vi "nanostage-init.vi"(3 "error in":errorcluster, 4 "Perform autozero?":bool=TRUE) -> (0 "error out":errorcluster, 2 "All conn. axes":string[](array[string]))   [LabVIEW 2017]
panel:
  out "USB: S/N out":string
  # "3D piezo nano stage"
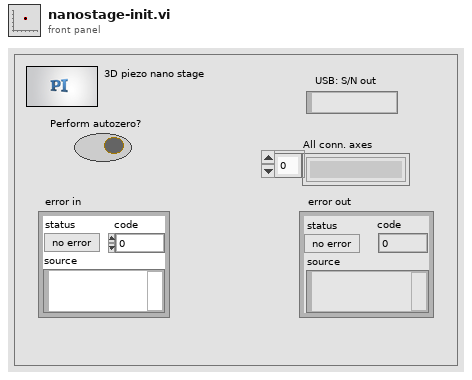
[diagram p1: front panel]
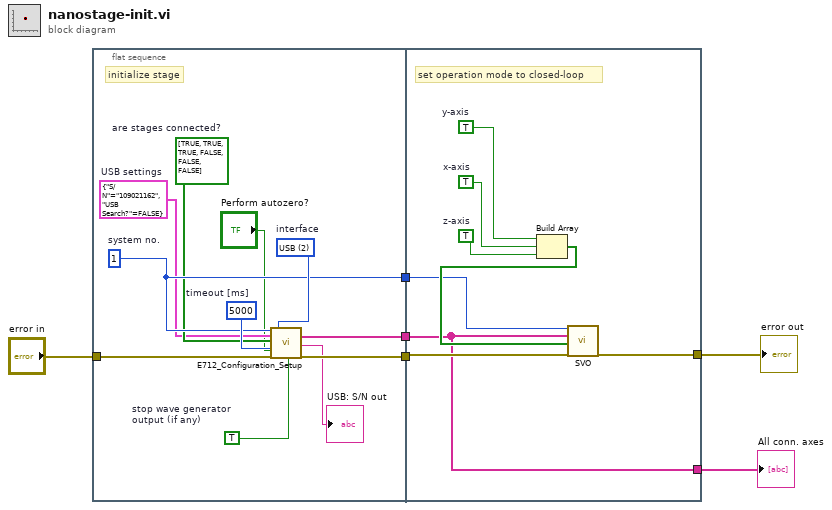
[diagram p0: block diagram]
diagram:
  n1 = flat-sequence {
    tunnel: [w15] -> w5
    tunnel: [w14] -> w4
    tunnel: [w9] -> w3
    tunnel: "error in" -> [w11]
    tunnel: w5 -> [w20]
    tunnel: w4 -> [w18]
    tunnel: w3 -> [w25]
    tunnel: [w19] -> w2
    tunnel: [w18] -> w1
    frame #0 {
      w10 = cluster{"S/N":string, "USB Search?":bool} {"S/N"="109021162", "USB Search?"=FALSE}  # USB settings
      w12 = bool[] [TRUE, TRUE, TRUE, FALSE, FALSE, FALSE]  # are stages connected?
      w13 = TRUE  # stop wave generator output (if any)
      w16 = 5000  # timeout [ms]
      w15 = 1  # system no.
      w17 = u16 2 items=["RS232", "TCP/IP", "USB"]  # interface
      # "initialize stage"
      n2 = call "E712_Configuration_Setup.vi"("System no."=w15, "USB settings"=w10, "Are stages connected?"=w12, "Perform autozero?"="Perform autozero?", "error in"=w11, "Interface"=w17, "Timeout"=w16, "Stop wave generator\noutput (if any)"=w13) -> ("All conn. axes"=w14:string[], "USB: S/N out"=→"USB: S/N out":string, "error out"=w9:errorcluster)  [unwired: 7 in, 2 out]
    }
    frame #1 {
      w21 = TRUE  # z-axis
      w22 = TRUE  # x-axis
      w23 = TRUE  # y-axis
      # "set operation mode to closed-loop"
      n3 = Build Array(w23, w22, w21) -> (w24:bool[])
      n4 = call "SVO.vi"("System no."=w20, "Axes to command"=w18, "Servo mode"=w24, "error in"=w25) -> ("error out"=w19:errorcluster)  [unwired: 15 in]
    }
  }
  "error out" <- w2
  "All conn. axes" <- w1
